vi "Write Field - Boolean.vi"(7 "field name":string, 8 "error in":errorcluster, 10 "value":bool, 11 "PV Data in":refnum<class "PV Data.lvclass">) -> (0 "error out":errorcluster, 2 "value out":bool, 3 "PV Data out":refnum<class "PV Data.lvclass">)   [LabVIEW 2020, in "PV Access.lvlib" / "PV Data.lvlib" / "PV Data.lvclass"]
uses:
  PV Data.lvclass
  PV Access.lvlib
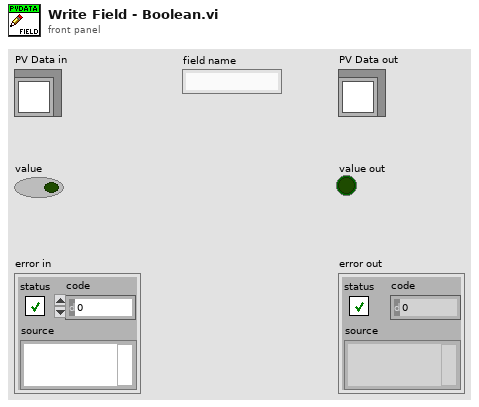
[diagram p1: front panel]
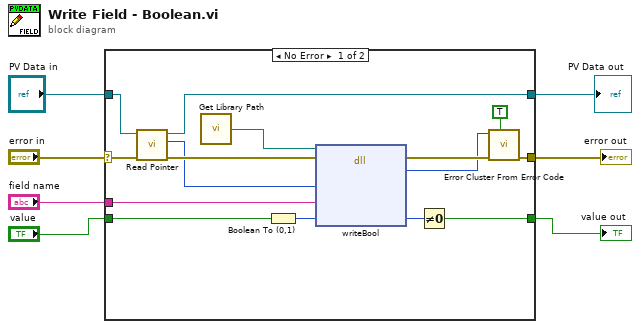
[diagram p0: block diagram]
diagram:
  n1 = case shown="No Error" "error in" {
    selector: "error in" -> [w14 w25]
    tunnel: [w16 w25] -> w7
    tunnel: "value" -> [w22 w24]
    tunnel: [w21 w24] -> w4
    tunnel: [w12 w23] -> w2
    tunnel: "PV Data in" -> [w15 w23]
    tunnel: "field name" -> [w10 _]
    frame No Error {
      n2 = call-dynamic "Read Pointer.vi"("error in (no error)"=w14, "Pointer Base in"=w15) -> ("error out"=w13:errorcluster, "Pointer"=w11:i64, "Pointer Base out"=w12:refnum<class "PV Data.lvclass">)  [unwired: 7 in]
      n3 = call "Get Library Path.vi"() -> ("Path"=w20:path)  [unwired: 1 in]
      n4 = Boolean To (0,1)(Boolean=w22) -> (0, 1=w9:i16)
      n5 = dll-call lib="?" fn="writeBool"(path in=w20, error in=w13, "value"=w11, "field_name"=w10, "new_value"=w9) -> (error out=w18:errorcluster, "err_code"=w17:i32, "new_value"=w8:i16)  [unwired: 3 in, 1 out]
      n6 = Not Equal To 0?(x=w8) -> (x != 0?=w21:bool)
      n7 = call <vilib>:"Error Cluster From Error Code.vi"("show call chain? (False)"=TRUE, "error in (no error)"=w18, "error code (0)"=w17) -> ("error out"=w16:errorcluster)  [unwired: 6 in]
    }
    frame Error {
    }
  }
  "error out" <- w7
  "value out" <- w4
  "PV Data out" <- w2
